vi "launch process ref bag.vi"(6 "launch items":T2, 7 "bag action":T1=enum."add", 11 "process ref IN":refnum<vi>) -> (3 "process ref OUT":refnum<vi>)   [LabVIEW 2020]
uses:
  launch items list.ctl
  que event bag action.ctl
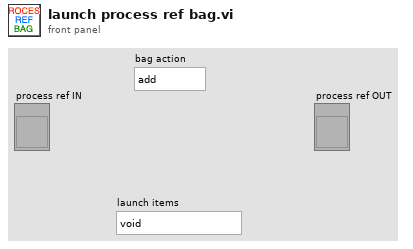
[diagram p1: front panel]
types:
  T1 = typedef "que event bag action.ctl" = enum16{"check", "add", "init"}
  T2 = typedef "launch items list.ctl" = enum16{"void", "source", "pll engine", "pll monitor", "sweeper engine", "sweeper monitor", "fitter"}
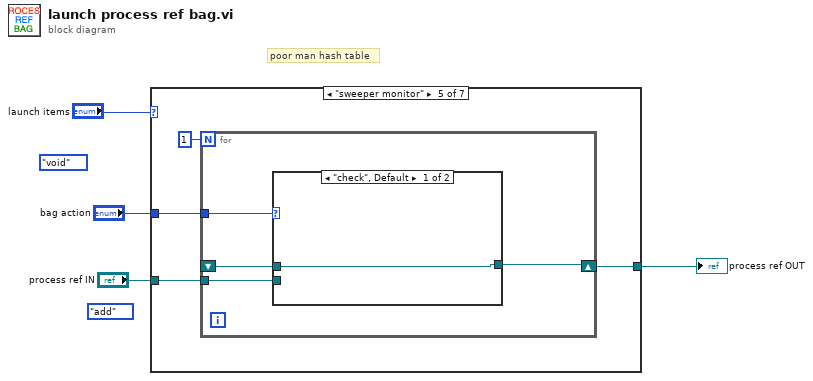
[diagram p0: block diagram]
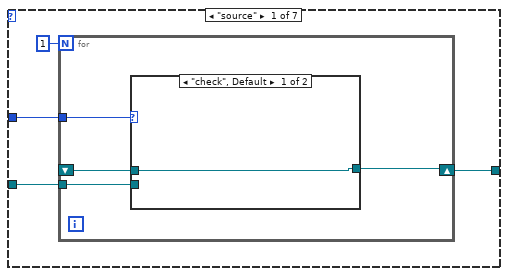
[diagram p2: hidden frame]
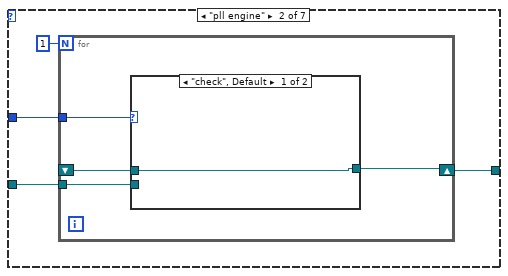
[diagram p4: hidden frame]
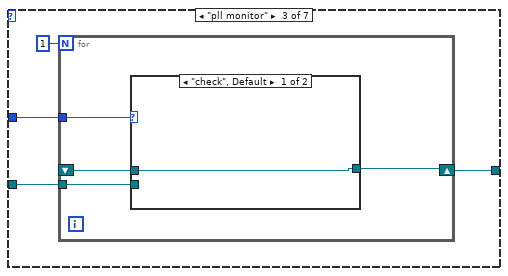
[diagram p6: hidden frame]
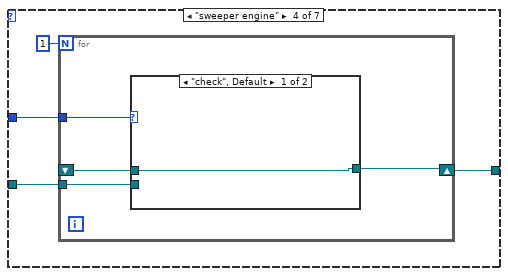
[diagram p8: hidden frame]
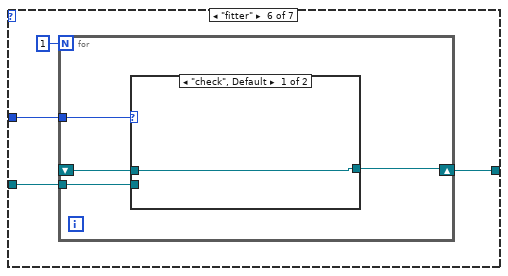
[diagram p11: hidden frame]
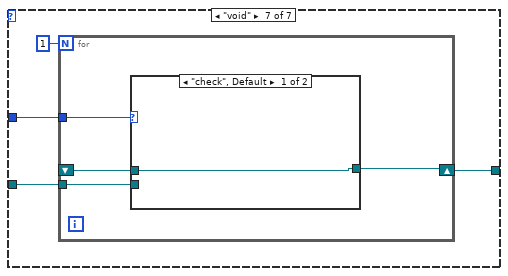
[diagram p13: hidden frame]
diagram:
  (unwired) que_event_bag_action."add" ("bag action")
  (unwired) launch_items_list."void" ("launch items")
  # "poor man hash table"
  n1 = case shown="\"sweeper monitor\"" "launch items" {
    tunnel: "process ref IN" -> [w7 w17 w27 w37 w47 w57 w67]
    tunnel: "bag action" -> [w6 w16 w26 w36 w46 w56 w66]
    tunnel: [w5 w15 w25 w35 w45 w55 w65] -> w1
    frame "source" {
      n2 = for {
        N: 1 -> [_]
        tunnel: w7 -> [w10]
        tunnel: w6 -> [w12]
        shift-right: [w11] -> w5
        shift-left: _ -> [w9]
        n3 = case shown="\"check\", Default" w12 {
          tunnel: [w13 w14] -> w11
          tunnel: w10 -> [_ w14]
          tunnel: w9 -> [w13 _]
          frame "check", Default {
          }
          frame "add" {
          }
        }
      }
    }
    frame "pll engine" {
      n4 = for {
        N: 1 -> [_]
        tunnel: w17 -> [w20]
        tunnel: w16 -> [w22]
        shift-right: [w21] -> w15
        shift-left: _ -> [w19]
        n5 = case shown="\"check\", Default" w22 {
          tunnel: [w23 w24] -> w21
          tunnel: w20 -> [_ w24]
          tunnel: w19 -> [w23 _]
          frame "check", Default {
          }
          frame "add" {
          }
        }
      }
    }
    frame "pll monitor" {
      n6 = for {
        N: 1 -> [_]
        tunnel: w27 -> [w30]
        tunnel: w26 -> [w32]
        shift-right: [w31] -> w25
        shift-left: _ -> [w29]
        n7 = case shown="\"check\", Default" w32 {
          tunnel: [w33 w34] -> w31
          tunnel: w30 -> [_ w34]
          tunnel: w29 -> [w33 _]
          frame "check", Default {
          }
          frame "add" {
          }
        }
      }
    }
    frame "sweeper engine" {
      n8 = for {
        N: 1 -> [_]
        tunnel: w37 -> [w40]
        tunnel: w36 -> [w42]
        shift-right: [w41] -> w35
        shift-left: _ -> [w39]
        n9 = case shown="\"check\", Default" w42 {
          tunnel: [w43 w44] -> w41
          tunnel: w40 -> [_ w44]
          tunnel: w39 -> [w43 _]
          frame "check", Default {
          }
          frame "add" {
          }
        }
      }
    }
    frame "sweeper monitor" {
      n10 = for {
        N: 1 -> [_]
        tunnel: w47 -> [w50]
        tunnel: w46 -> [w52]
        shift-right: [w51] -> w45
        shift-left: _ -> [w49]
        n11 = case shown="\"check\", Default" w52 {
          tunnel: [w53 w54] -> w51
          tunnel: w50 -> [_ w54]
          tunnel: w49 -> [w53 _]
          frame "check", Default {
          }
          frame "add" {
          }
        }
      }
    }
    frame "fitter" {
      n12 = for {
        N: 1 -> [_]
        tunnel: w57 -> [w60]
        tunnel: w56 -> [w62]
        shift-right: [w61] -> w55
        shift-left: _ -> [w59]
        n13 = case shown="\"check\", Default" w62 {
          tunnel: [w63 w64] -> w61
          tunnel: w60 -> [_ w64]
          tunnel: w59 -> [w63 _]
          frame "check", Default {
          }
          frame "add" {
          }
        }
      }
    }
    frame "void" {
      n14 = for {
        N: 1 -> [_]
        tunnel: w67 -> [w70]
        tunnel: w66 -> [w72]
        shift-right: [w71] -> w65
        shift-left: _ -> [w69]
        n15 = case shown="\"check\", Default" w72 {
          tunnel: [w73 w74] -> w71
          tunnel: w70 -> [_ w74]
          tunnel: w69 -> [w73 _]
          frame "check", Default {
          }
          frame "add" {
          }
        }
      }
    }
  }
  "process ref OUT" <- w1
